vi "LabViewPidSimple.vi"() -> ()   [LabVIEW 2018, in "Pid.lvlib"]
uses:
  Pid.lvlib
  <vilib>/Platform/TimedLoop/XDataNode/timing_clust.ctl
  <vilib>/Platform/TimedLoop/XDataNode/nitl_modes.ctl
  <vilib>/Platform/TimedLoop/XDataNode/wakeup.ctl
  <vilib>/addons/control/pid/autopid.llb/PID autotuning parameters (FO).ctl
  <vilib>/addons/control/pid/pid.llb/PID (DBL).vi
  <vilib>/platform/TimedLoop/XDataNode/XDataNode.xnode
  <vilib>/Platform/TimedLoop/XDataNode/XDNodeRunTimeDep.lvlib
  <vilib>/addons/control/pid/NI_PID_autopid.lvlib
  <vilib>/addons/control/pid/NI_PID_pid.lvlib
panel:
  out "Loop and out":errorcluster
  out "Modbus":errorcluster
  out "File":errorcluster
  in  "Setpoint":dbl(slide) scale=0.0..255.0
  in  "Manual":dbl(slide) scale=0.0..255.0
  in  "Start tunning":bool
  in  "On/Off":bool
  out "Temperature":dbl(slide) scale=0.0..255.0
  out "Output":dbl(knob) scale=0.0..255.0
  in  "Stop":bool
  out "Off Hook":bool
  out "Communication Failure":bool
  out "Updating":bool
  in  "Frequency":dbl(slide) scale=1.0..100.0
  out "Interval":i64
  out "Counter":i32
  out "Time (ms)":u32
  out "Tun Delay time (s)":dbl
  out "Tun Time constant (s)":dbl
  out "Tun Process gain":dbl
  out "Tun Td":dbl
  out "Tun Ti":dbl
  out "Tun Kp":dbl
  out "Tunning":bool
  in  "Auto/Manual":bool
  in  "Beta":dbl
  in  "Alfa":dbl
  in  "Type":enum16{"P", "PI", "PID"}(ring)
  in  "Step amplitude":dbl
  in  "Time constant factor":dbl
  in  "Reset Tune":bool
  in  "Delay time (s)":dbl
  in  "Time constant (s)":dbl
  in  "Process gain":dbl
  out "Tunning Complete":bool
  out "dt PID":dbl
  in  "Reset PID":bool
  out "dt loop":dbl
  out "Single Update (Multiple Plots, stacked)":T1(graph)
  out "Kd":sgl
  out "Ki":sgl
  in  "Set Kp":sgl
  in  "Set Td":sgl
  in  "Set Ti":sgl
  in  "Apply Max time":bool
  in  "Scale":bool
  in  "Max time":dbl
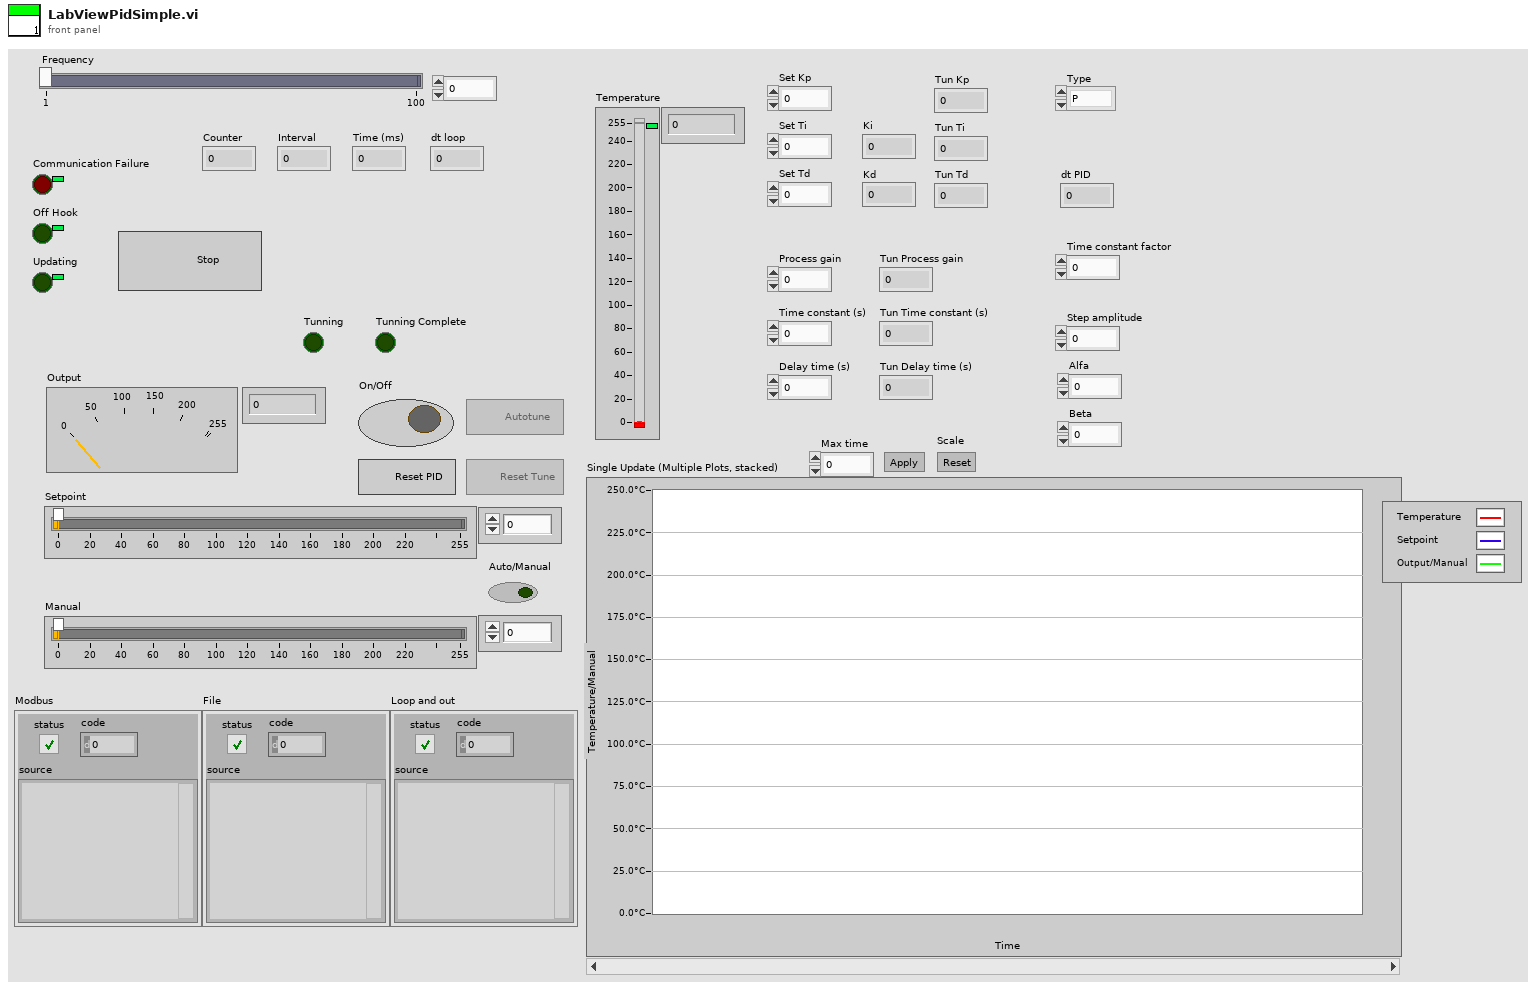
[diagram p1: front panel]
types:
  T1 = cluster{"Temperature":dbl, "Setpoint":dbl, "output":dbl}
  T2 = typedef "XDNodeRunTimeDep.lvlib/timing_clust.ctl" = cluster{"Expected End [f-1]":u64, "Actual End [f-1]":u64, "Finished Late? [f-1]":bool, "Expected End [i-1]":u64, "Actual End [i-1]":u64, "Finished Late? [i-1]":bool, "Expected Start [i]":u64, "Actual Start [i]":u64, "Expected Start [f]":u64, "Actual Start [f]":u64, "Source Name":string, "Structure Name":string, "Period":i64, "Deadline":i64, "Offset":i64, "Start":i64, "Priority":i32, "Timeout":i32, "Mode":T3, "Wakeup Reason":T4, "Error":errorcluster, "Source Type":string, "Secondary Source Type":string, "Global End Time":u64, "Global Start Time":u64, "Frame Duration":u64, "Iteration Duration":u64, "Assigned CPU":i32, "I/O Scan Engine Mode":u32}
  T3 = typedef "XDNodeRunTimeDep.lvlib/nitl_modes.ctl" = enum32{"No Change", "Process missed periods, maintain original phase", "Discard missed periods, maintain original phase", "Process missed periods, ignore original phase", "Discard missed periods, ignore original phase"}
  T4 = typedef "XDNodeRunTimeDep.lvlib/wakeup.ctl" = enum32{"Normal", "Aborted", "Asynchronous wakeup", "Timing source error", "Timed loop error", "Timeout"}
  T5 = typedef "NI_PID_autopid.lvlib/PID autotuning parameters (FO).ctl" = cluster{"type of controller":u16, "time constant factor":dbl, "step amplitude":dbl}
  T6 = cluster{"process gain":dbl, "time constant (s)":dbl, "delay time (s)":dbl}
  T7 = cluster{"proportional gain (Kc)":dbl, "integral time (Ti, min)":dbl, "derivative time (Td, min)":dbl}
  T8 = cluster{"Temperature":dbl, "Setpoint":dbl, "Manual":dbl}
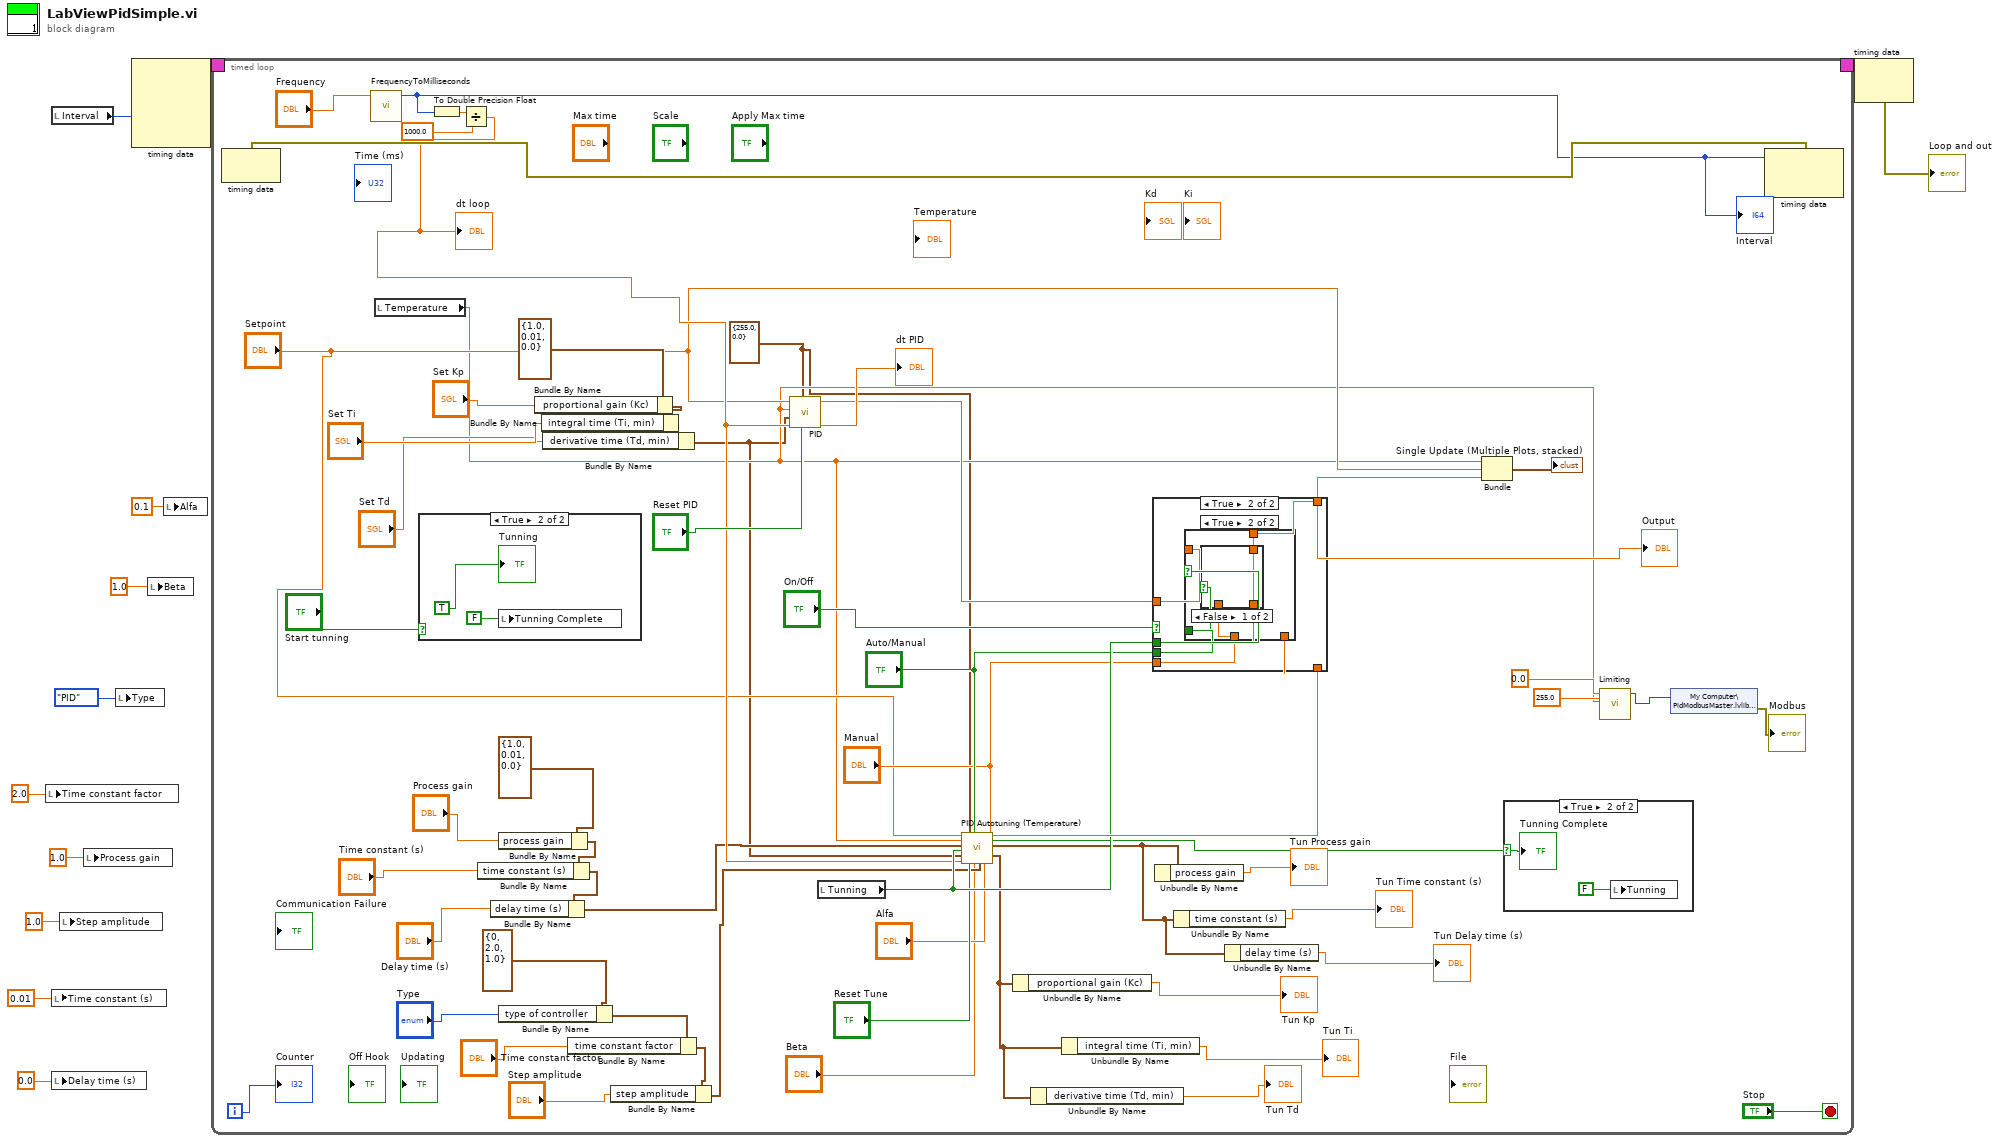
[diagram p0: block diagram]
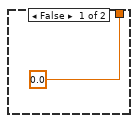
[diagram p4: hidden frame]
diagram:
  n1 = local write "Time constant factor"(2.0 ("Time constant factor")) -> ()
  n2 = local read "Interval"() -> (w10:i64)
  n3 = local write "Time constant (s)"(0.01 ("Time constant (s)")) -> ()
  n4 = local write "Delay time (s)"(0.0 ("Delay time (s)")) -> ()
  n5 = local write "Step amplitude"(1.0 ("Step amplitude")) -> ()
  n6 = local write "Process gain"(1.0 ("Process gain")) -> ()
  n7 = local write "Type"(enum16{"P", "PI", "PID"}."PID" ("Type")) -> ()
  n8 = node-c288(w10) -> (w12:T2)  [unwired: 3 in]
  n9 = local write "Beta"(1.0 ("beta")) -> ()
  n10 = local write "Alfa"(0.1 ("alpha")) -> ()
  n11 = timed-loop {
    timing: w12 -> [_]
    timing-out: [_] -> w11
    i -> [w61]
    stop <- "Stop" stop-if-true
    w37 = cluster{"output high":dbl, "output low":dbl} {"output high"=255.0, "output low"=0.0} ("output range")
    n12 = node-c288() -> (w71:errorcluster)  [unwired: 1 in]
    n13 = call "FrequencyToMilliseconds.vi"("Frequency"="Frequency") -> ("Numeric"=w44:i64)  [unwired: 10 in]
    "Interval" <- w44
    n14 = local read "Temperature"() -> (w38:dbl)
    n15 = case shown="True" "Start tunning" {
      frame False {
      }
      frame True {
        n16 = local write "Tunning Complete"(FALSE ("Tunning Complete")) -> ()
        "Tunning" <- TRUE
      }
    }
    n17 = To Double Precision Float(number=w44) -> (double precision float=w43:dbl)
    n18 = Divide(x=w43, y=1000.0) -> (x/y=w41:dbl)
    "dt loop" <- w41
    n19 = Bundle By Name(cluster=T6 {"process gain"=1.0, "time constant (s)"=0.01, "delay time (s)"=0.0} ("plant parameters in"), "process gain"="Process gain") -> (w28:T6)
    n20 = Bundle By Name(cluster=w28, "time constant (s)"="Time constant (s)") -> (w27:T6)
    n21 = Bundle By Name(cluster=w27, "delay time (s)"="Delay time (s)") -> (w26:T6)
    n22 = Bundle By Name(cluster=T5 {"type of controller"=0, "time constant factor"=2.0, "step amplitude"=1.0} ("autotuning parameters"), "type of controller"="Type") -> (w34:T5)
    n23 = Bundle By Name(cluster=T7 {"proportional gain (Kc)"=1.0, "integral time (Ti, min)"=0.01, "derivative time (Td, min)"=0.0} ("PID gains"), "proportional gain (Kc)"="Set Kp") -> (w69:T7)
    n24 = Bundle By Name(cluster=w69, "integral time (Ti, min)"="Set Ti") -> (w68:T7)
    n25 = Bundle By Name(cluster=w68, "derivative time (Td, min)"="Set Td") -> (w25:T7)
    n26 = Bundle By Name(cluster=w34, "time constant factor"="Time constant factor") -> (w33:T5)
    n27 = Bundle By Name(cluster=w33, "step amplitude"="Step amplitude") -> (w32:T5)
    n28 = call-poly <vilib>:"PID.vi"("reinitialize? (F)"="Reset PID", "output range"=w37, "dt (s)"=w41, "PID gains"=w25, "process variable"=w38, "setpoint"="Setpoint") -> ("dt out (s)"=→"dt PID":dbl, "output"=w57:dbl)  [unwired: 4 in]
    n29 = local read "Tunning"() -> (w49:bool)
    n30 = call <vilib>:"PID Autotuning (Temperature).vi"("desired temperature"="Setpoint", "measured temperature"=w38, "plant parameters in"=w26, "autotune? (F)"=w49, "PID gains in"=w25, "dt (s)"=w41, "output range"=w37, "reinitialize? (F)"="Reset Tune", "auto? (T)"="Auto/Manual", "beta"="Beta", "manual control"="Manual", "autotuning parameters"=w32, "alpha"="Alfa") -> ("output"=w50:dbl, "tuning completed?"=w47:bool, "plant parameters out"=w22:T6, "PID gains out"=w24:T7)  [unwired: 3 in]
    n31 = Unbundle By Name(w24) -> ("proportional gain (Kc)"=→"Tun Kp":dbl)
    n32 = Unbundle By Name(w24) -> ("derivative time (Td, min)"=→"Tun Td":dbl)
    n33 = Unbundle By Name(w24) -> ("integral time (Ti, min)"=→"Tun Ti":dbl)
    n34 = case shown="True" "On/Off" {
      tunnel: [0.0 w80] -> w58
      tunnel: w57 -> [_ w79]
      tunnel: w49 -> [_ w82]
      tunnel: w50 -> [_ w81]
      tunnel: "Auto/Manual" -> [_ w78]
      tunnel: "Manual" -> [_ w77]
      frame False {
      }
      frame True {
        n35 = case shown="True" w82 {
          tunnel: [w83 w85] -> w80
          tunnel: w81 -> [_ w84]
          tunnel: w79 -> [w83 _]
          tunnel: w78 -> [_ w87]
          tunnel: w77 -> [_ w86]
          frame False {
          }
          frame True {
            n36 = case shown="False" w87 {
              tunnel: w86 -> [_ w89]
              tunnel: [w88 w89] -> w85
              tunnel: w84 -> [w88 _]
              frame False {
              }
              frame True {
              }
            }
          }
        }
      }
    }
    "Output" <- w58
    n37 = Unbundle By Name(w22) -> ("process gain"=→"Tun Process gain":dbl)
    n38 = Unbundle By Name(w22) -> ("time constant (s)"=→"Tun Time constant (s)":dbl)
    n39 = Unbundle By Name(w22) -> ("delay time (s)"=→"Tun Delay time (s)":dbl)
    n40 = Bundle("Temperature"=w38, "Setpoint"="Setpoint", "Manual"=w58) -> (→"Single Update (Multiple Plots, stacked)":T8)  [unwired: 1 in]
    n41 = case shown="True" w47 {
      selector: w47 -> [_ w73]
      frame False {
      }
      frame True {
        n42 = local write "Tunning"(FALSE ("Tunning")) -> ()
        "Tunning Complete" <- w73
      }
    }
    n43 = call "Limiting.vi"("Maximum"=255.0 ("y"), "Value"=w38, "Minimum"=0.0 ("y")) -> ("Output"=w53:i16)  [unwired: 8 in]
    n44 = shared-variable "My Computer\\PidModbusMaster.lvlib\\S400001"(w53) -> (error out=→"Modbus":errorcluster)  [unwired: 1 in]
    n45 = node-c288(w71, w44) -> ()  [unwired: 1 out]
    "Counter" <- w61
  }
  n46 = node-c288(w11) -> (→"Loop and out":errorcluster)
